vi "TestExec.Process Options for Archive Summary UUT Folder.vi"(9 "Args":string[](array[string]), 10 "ArchiveDir":path, 11 "UUTDir":path) -> (0 "Error":errorcluster, 1 "Destination Files":path[](array[path]), 2 "Source Files":path[](array[path]), 3 "Destination Path":path)   [LabVIEW 2018]
uses:
  <vilib>/KATE/Files/File Utils.lvlib
panel:
  # "ArchiveSumUUTData(SubFolder1, Subfolder2, . . ., FileInfoDelim, Pattern1, SubFolder1, AppendSNTime1, Pattern2, SubFolder2, AppendSNTime2, ...)\n  FileInfoDelim\n    The FilePattern Delimiter is the key word: \"FileInfo\"\n    All arguments after this delimiter are file pattern information\n \n  FileInfo\n    The file info has 3 parts:\n       1) SearchPattern\n           These are file search patterns similar to the matching used in matching wildcards in Windows \n            Example Patterns: \"*.csv\", \"*.jpg\"\n            Since commas are used as argument delimiters, a coma cannot be used in the pattern.     \n        2) SubFolder\n           This is the subfolder these files are to be put into.\n            If this is empty, the files will be put into the root folder.\n        3) Append SN Time\n            If this is TRUE or 1, the SN and Time of the UUTDir will be appended to the file name.\n            If this is any value but True or 1, empty, the files will be put into the root folder.\n\n    \nExample:\nThe following example will copy all CSV and JPG files to the \nArchiveUUTData($Mode, $Date, FilePatterns, *.csv, *.jpg)"
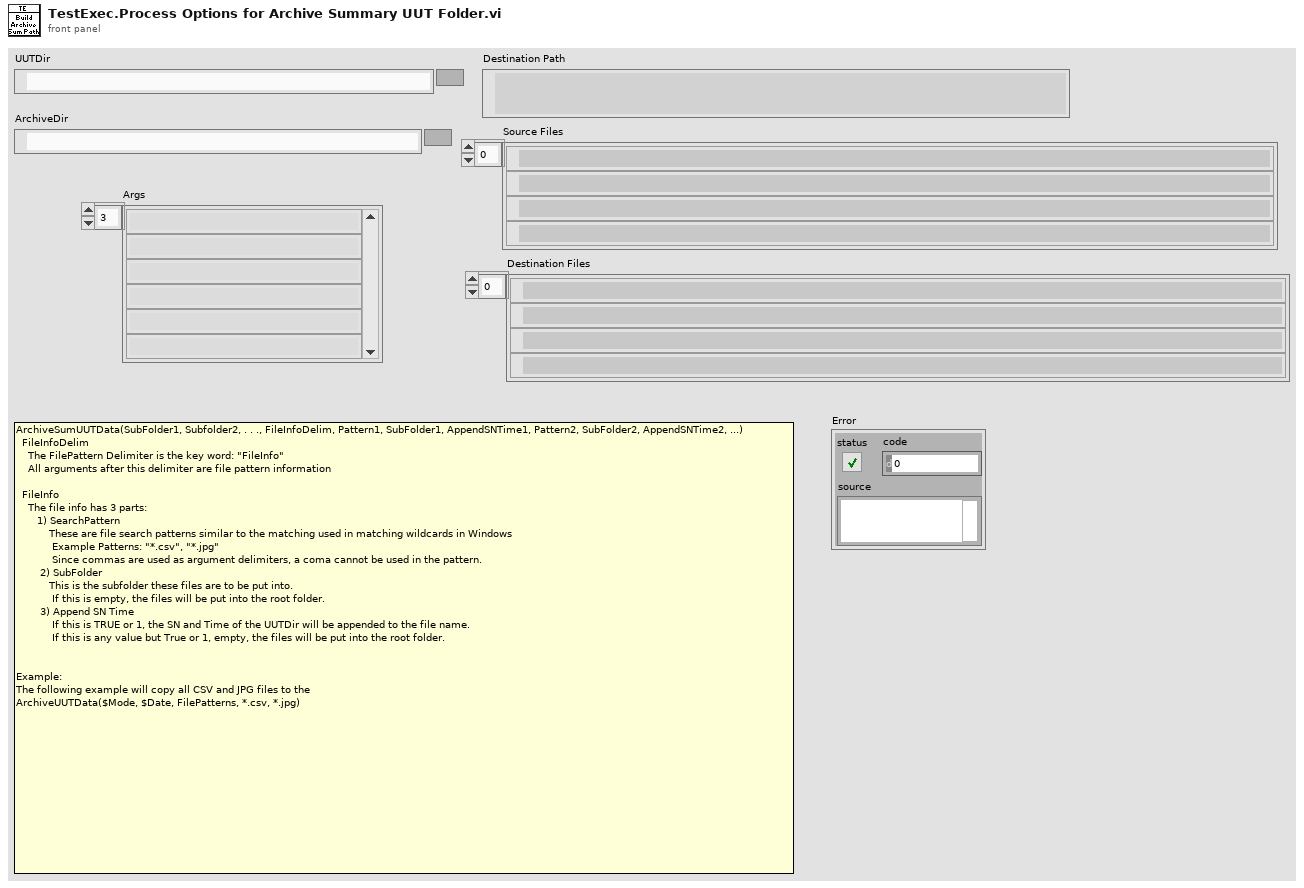
[diagram p1: front panel]
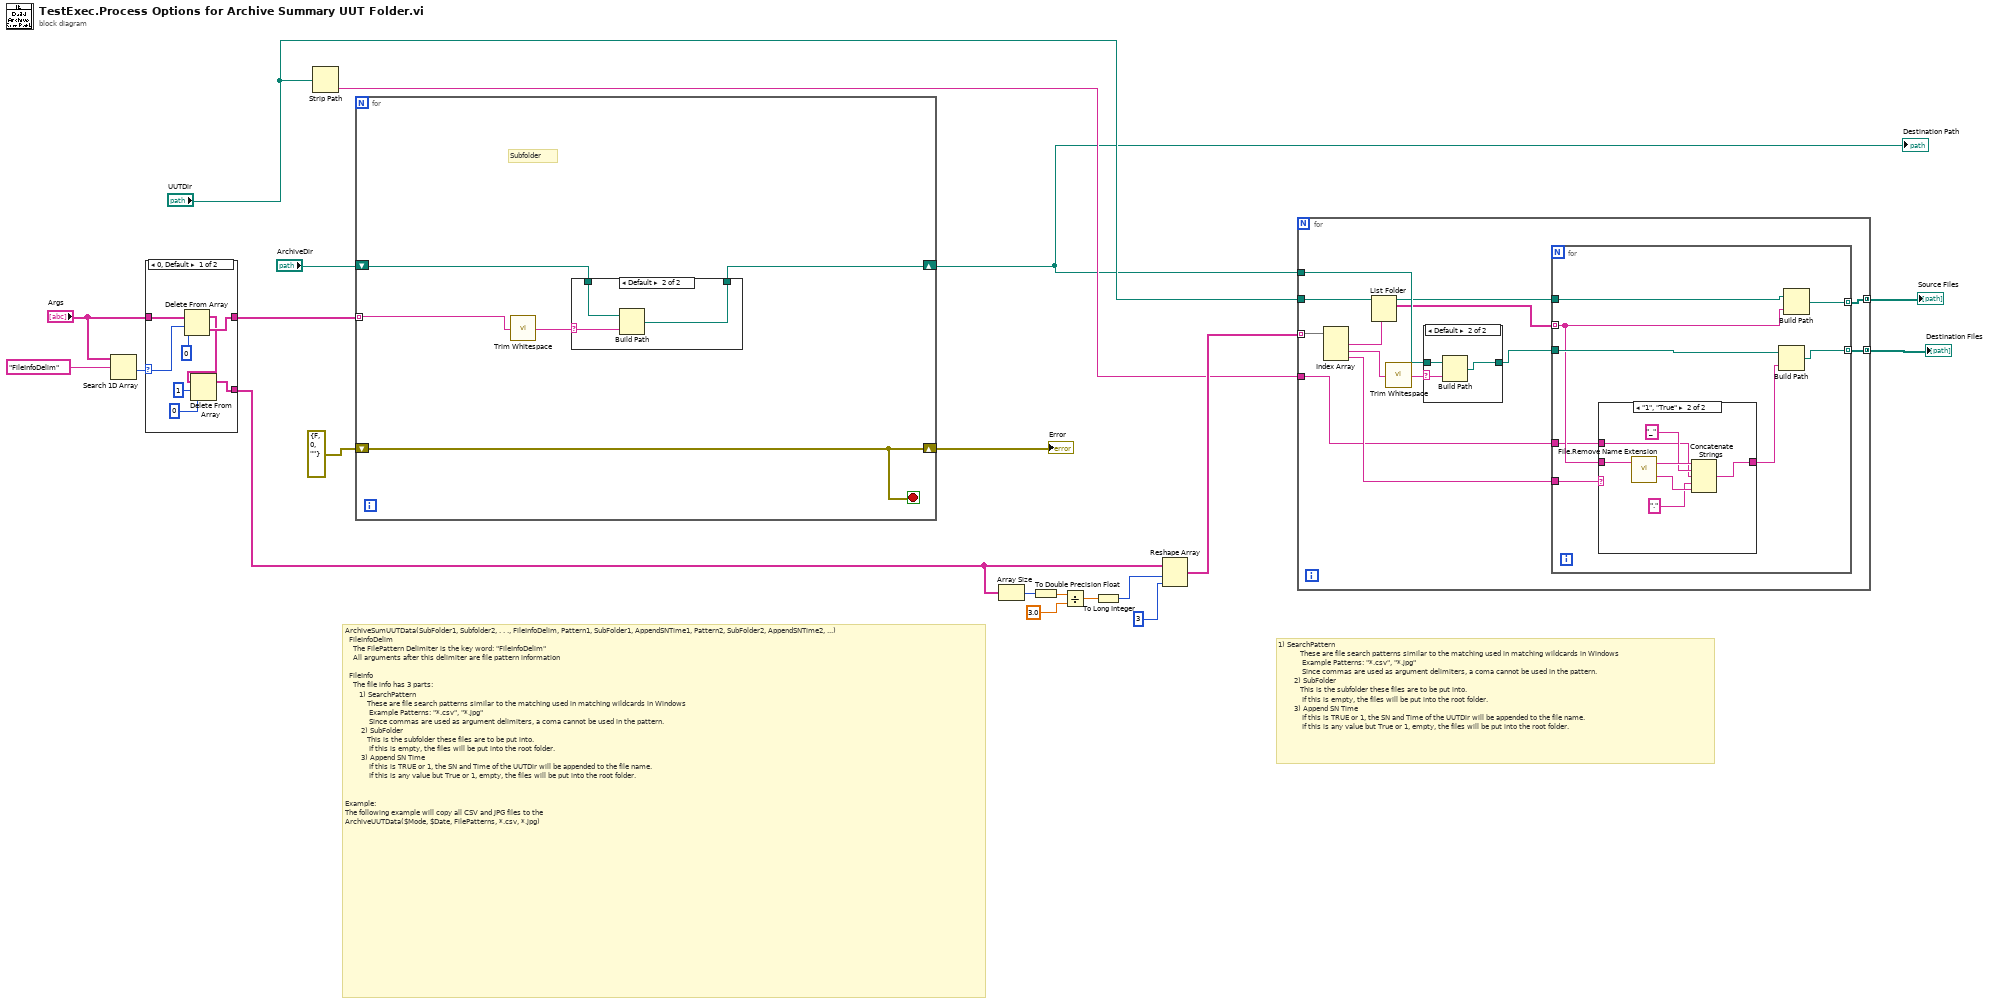
[diagram p0: block diagram]
diagram:
  # "1) SearchPattern\n           These are file search patterns similar to the matching used in matching wildcards in Windows \n            Example Patterns: \"*.csv\", \"*.jpg\"\n            Since commas are used as argument delimiters, a coma cannot be used in the pattern.     \n        2) SubFolder\n           This is the subfolder these files are to be put into.\n            If this is empty, the files will be put into the root folder.\n        3) Append SN Time\n            If this is TRUE or 1, the SN and Time of the UUTDir will be appended to the file name.\n            If this is any value but True or 1, empty, the files will be put into the root folder."
  # "ArchiveSumUUTData(SubFolder1, Subfolder2, . . ., FileInfoDelim, Pattern1, SubFolder1, AppendSNTime1, Pattern2, SubFolder2, AppendSNTime2, ...)\n  FileInfoDelim\n    The FilePattern Delimiter is the key word: \"FileInfoDelim\"\n    All arguments after this delimiter are file pattern information\n \n  FileInfo\n    The file info has 3 parts:\n       1) SearchPattern\n           These are file search patterns similar to the matching used in matching wildcards in Windows \n            Example Patterns: \"*.csv\", \"*.jpg\"\n            Since commas are used as argument delimiters, a coma cannot be used in the pattern.     \n        2) SubFolder\n           This is the subfolder these files are to be put into.\n            If this is empty, the files will be put into the root folder.\n        3) Append SN Time\n            If this is TRUE or 1, the SN and Time of the UUTDir will be appended to the file name.\n            If this is any value but True or 1, empty, the files will be put into the root folder.\n\n    \nExample:\nThe following example will copy all CSV and JPG files to the \nArchiveUUTData($Mode, $Date, FilePatterns, *.csv, *.jpg)"
  n1 = Search 1D Array(1D array="Args", element="FileInfoDelim") -> (index of element=w16:i32)  [unwired: 1 in]
  n2 = case shown="0, Default" w16 {
    selector: w16 -> [w26 _]
    tunnel: "Args" -> [w28 w29]
    tunnel: [w27 w29] -> w14
    tunnel: [w21 _] -> w13
    frame 0, Default {
      n3 = Delete From Array(array=w28, length=w26, index=0) -> (deleted portion=w27:string[], array with subset deleted=w24:string[])
      n4 = Delete From Array(array=w24, length=1, index=0) -> (array with subset deleted=w21:string[])  [unwired: 1 out]
    }
    frame -1 {
    }
  }
  n5 = Strip Path(path="UUTDir") -> (name=w3:string)  [unwired: 1 out]
  n6 = for {
    tunnel: w14 -> [w31] mode=indexing
    shift-right: [w33] -> w1
    shift-left: "ArchiveDir" -> [w34]
    shift-right: [w32] -> w18
    shift-left: errorcluster {"status"=FALSE, "code"=0, "source"=""} ("error constant") -> [w32]
    stop <- w32 stop-if-true
    # "Subfolder"
    n7 = call <vilib>:"Trim Whitespace.vi"("string"=w31) -> ("trimmed string"=w30:string)  [unwired: 1 in]
    n8 = case shown="Default" w30 {
      selector: w30 -> [_ w38]
      tunnel: w34 -> [w35 w37]
      tunnel: [w35 w36] -> w33
      frame "" {
      }
      frame Default {
        n9 = Build Path(base path=w37, name or relative path=w38) -> (appended path=w36:path)
      }
    }
  }
  "Destination Path" <- w1
  "Error" <- w18
  n10 = Array Size(array=w13) -> (size(s)=w12:i32)
  n11 = To Double Precision Float(number=w12) -> (double precision float=w11:dbl)
  n12 = Divide(x=w11, y=3.0) -> (x/y=w9:dbl)
  n13 = To Long Integer(number=w9) -> (32bit integer=w8:i32)
  n14 = Reshape Array(w13, w8, 3) -> (w6:string[][])
  n15 = for {
    tunnel: w6 -> [w51] mode=indexing
    tunnel: "UUTDir" -> [w49]
    tunnel: [w41] -> w4 mode=concatenating
    tunnel: w1 -> [w48]
    tunnel: w3 -> [w39]
    tunnel: [w40] -> w2 mode=concatenating
    n16 = Index Array(array=w51) -> (element #1=w50:string, element #2=w47:string, element #3=w45:string)  [unwired: 3 in]
    n17 = List Folder(path=w49, pattern=w50) -> (path out=w44:path, filenames=w42:string[])  [unwired: 2 in, 2 out]
    n18 = call <vilib>:"Trim Whitespace.vi"("string"=w47) -> ("trimmed string"=w46:string)  [unwired: 1 in]
    n19 = case shown="Default" w46 {
      selector: w46 -> [_ w70]
      tunnel: w48 -> [w68 w71]
      tunnel: [w68 w69] -> w43
      frame "" {
      }
      frame Default {
        n20 = Build Path(base path=w71, name or relative path=w70) -> (appended path=w69:path)
      }
    }
    n21 = for {
      tunnel: w45 -> [w59]
      tunnel: w44 -> [w57]
      tunnel: w43 -> [w56]
      tunnel: w42 -> [w55] mode=indexing
      tunnel: [w54] -> w41 mode=indexing
      tunnel: [w53] -> w40 mode=indexing
      tunnel: w39 -> [w52]
      n22 = case shown="\"1\", \"True\"" w59 {
        tunnel: w55 -> [w60 w67]
        tunnel: [w60 w63] -> w58
        tunnel: w52 -> [_ w64]
        frame "False", Default {
        }
        frame "1", "True" {
          n23 = call <vilib>:"File.Remove Name Extension.vi"("File Name"=w67) -> ("Ext"=w62:string, "Name Less Ext"=w66:string)  [unwired: 1 in]
          n24 = Concatenate Strings(w66, "_", w64, ".", w62) -> (w63:string)
        }
      }
      n25 = Build Path(base path=w56, name or relative path=w58) -> (appended path=w53:path)
      n26 = Build Path(base path=w57, name or relative path=w55) -> (appended path=w54:path)
    }
  }
  "Destination Files" <- w2
  "Source Files" <- w4
